vi "Update_AM.vi"(7 "AM Modulation Mode Cluster":T2={"waveform (1: Sine)"=1, "Depth (%)"=50.0, "Modulation source"=0, "AM Frequency (Hz)"=10.0, "ON/OFF"=FALSE} {"Modulation source" items=["Intern", "Extern"]; "waveform (1: Sine)" items=["Sine"=1, "Square"=2, "Pulse"=1002, "Ramp"=1001, "Noise"=1003, "DC"=6, "Sin(x)/x"=1004, "Gaussian"=1005, "Lorentz"=1006, "Exponential Rise"=1007, "Exponential Decay"=1008, "Haversine"=1009]}, 8 "error in (no error)":errorcluster {"code" format="%.0x"}, 10 "channel name (\"1\")":string="1", 11 "resource name":refnum<k15>) -> (0 "error out":errorcluster, 1 "output cluster":T1, 3 "instrument handle out":refnum<k15>)   [LabVIEW 2015, in "MyToolsFunction.lvlib"]
uses:
  ICcamera/MyToolsFunction.lvlib
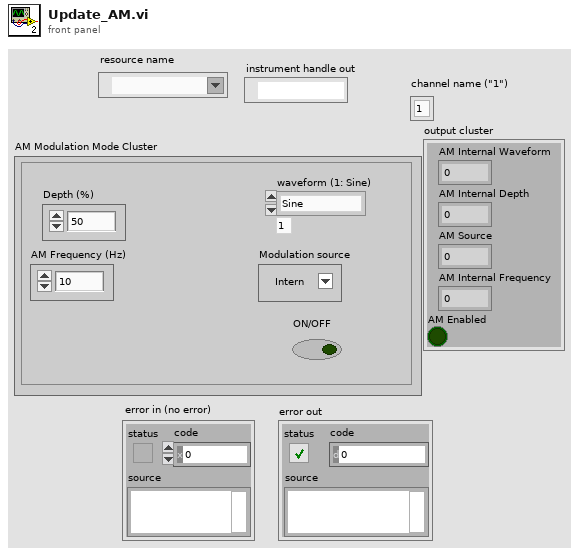
[diagram p1: front panel]
types:
  T1 = cluster{"AM Internal Waveform":i32, "AM Internal Depth":dbl, "AM Source":i32, "AM Internal Frequency":dbl, "AM Enabled":bool}
  T2 = cluster{"waveform (1: Sine)":i32, "Depth (%)":dbl, "Modulation source":u16, "AM Frequency (Hz)":dbl, "ON/OFF":bool}
  T3 = cluster{"FM Internal Waveform By Channel":i32, "FM Deviation By Channel":dbl, "AM Source":i32, "AM Internal Frequency By Channel":dbl, "AM Enabled":bool}
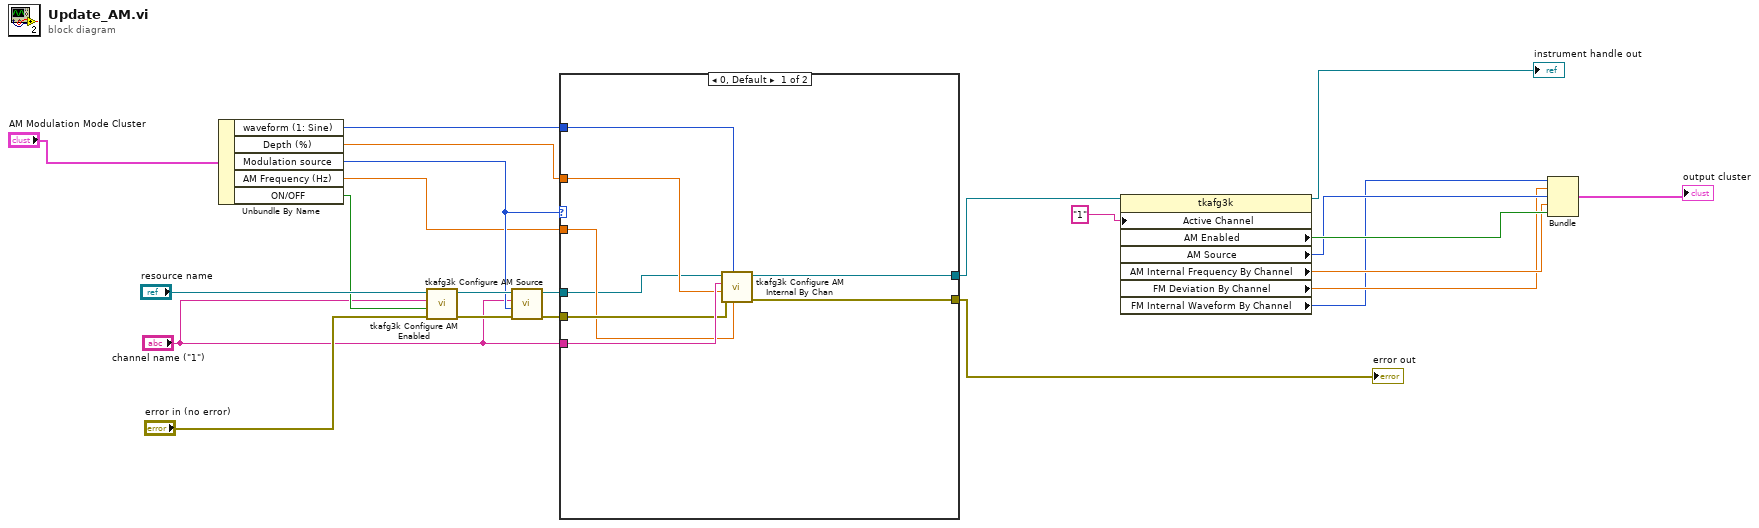
[diagram p0: block diagram]
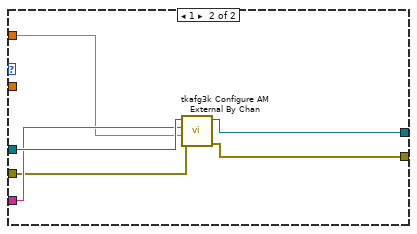
[diagram p2: hidden frame]
diagram:
  n1 = Unbundle By Name("AM Modulation Mode Cluster") -> ("waveform (1: Sine)"=w12:i32, "Depth (%)"=w14:dbl, "Modulation source"=w18:u16, "AM Frequency (Hz)"=w13:dbl, "ON/OFF"=w22:bool)
  n2 = call <instrlib>:"tkafg3k Configure AM Enabled.vi"("error in (no error)"="error in (no error)", "AM enabled (True)"=w22, "channel name (\"1\")"="channel name (\"1\")", "instrument handle"="resource name") -> ("error out"=w19:errorcluster, "instrument handle out"=w20:refnum<k15>)  [unwired: 6 in]
  n3 = call <instrlib>:"tkafg3k Configure AM Source.vi"("error in (no error)"=w19, "source (0: Internal)"=w18, "channel name (\"1\")"="channel name (\"1\")", "instrument handle"=w20) -> ("error out"=w16:errorcluster, "instrument handle out"=w17:refnum<k15>)  [unwired: 6 in]
  n4 = case shown="0, Default" w18 {
    tunnel: w17 -> [w24 w37]
    tunnel: w16 -> [w30 w34]
    tunnel: "channel name (\"1\")" -> [w31 w36]
    tunnel: w14 -> [w29 w35]
    tunnel: w13 -> [w28 _]
    tunnel: [w27 w33] -> w11
    tunnel: [w26 w32] -> w1
    tunnel: w12 -> [w25 _]
    frame 0, Default {
      n5 = call <instrlib>:"tkafg3k Configure AM Internal By Chan.vi"("Modulation Frequency (10000.0)"=w28, "Modulation Waveform (1: Sine)"=w25, "error in (no error)"=w30, "Modulation Depth (50.0)"=w29, "Channel Name (\"1\")"=w31, "instrument handle"=w24) -> ("error out"=w27:errorcluster, "instrument handle out"=w26:refnum<k15>)  [unwired: 4 in]
    }
    frame 1 {
      n6 = call <instrlib>:"tkafg3k Configure AM External By Chan.vi"("error in (no error)"=w34, "Modulation Depth (50.0)"=w35, "Channel Name (\"1\")"=w36, "instrument handle"=w37) -> ("error out"=w33:errorcluster, "instrument handle out"=w32:refnum<k15>)  [unwired: 6 in]
    }
  }
  "error out" <- w11
  n7 = property class="tkafg3k"(reference=w1, "Active Channel"="1") -> (reference out=→"instrument handle out":refnum<k15>, "AM Enabled"=w7:bool, "AM Source"=w6:i32, "AM Internal Frequency By Channel"=w5:dbl, "FM Deviation By Channel"=w3:dbl, "FM Internal Waveform By Channel"=w2:i32)  [unwired: 1 in, 1 out]
  n8 = Bundle("FM Internal Waveform By Channel"=w2, "FM Deviation By Channel"=w3, "AM Source"=w6, "AM Internal Frequency By Channel"=w5, "AM Enabled"=w7) -> (→"output cluster":T3)  [unwired: 1 in]
